vi "Unbundle.vi"(11 "Cluster":T1) -> (1 "String":string, 2 "Boolean":bool, 3 "Gauge":dbl(knob) scale=0.0..10.0)   [LabVIEW 2024]
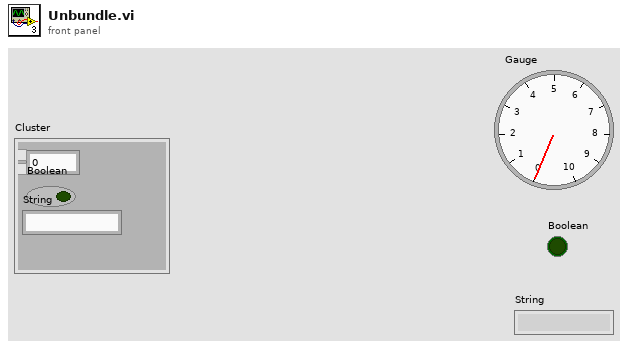
[diagram p1: front panel]
types:
  T1 = cluster{"Numeric":dbl, "Boolean":bool, "String":string}
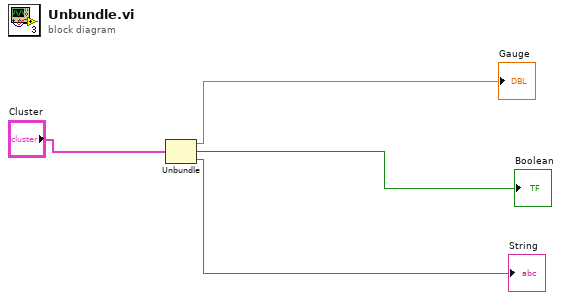
[diagram p0: block diagram]
diagram:
  n1 = Unbundle("Cluster") -> ("Numeric"=→"Gauge":dbl, "Boolean"=→"Boolean":bool, "String"=→"String":string)
